vi "Gadgeton.vi"() -> ()   [LabVIEW 2019]
uses:
  <userlib>/_SmartBalloon/Balloon Generic/Aesthetics.ctl
  <userlib>/_SmartBalloon/API/Read Events.vi
  <userlib>/_SmartBalloon/Symbol Text Balloon/Symbol Text Balloon.lvclass
  C:/Program Files (x86)/National Instruments/LabVIEW 2019/user.lib/_SmartBalloon/Balloon Generic/Balloon.lvclass
  <vilib>/Utility/inputDevices.llb/closeKeyboard.vi
  <vilib>/Utility/inputDevices.llb/keyboardAcquire.vi
  <vilib>/Utility/inputDevices.llb/mouseAcquire.vi
  <vilib>/Utility/inputDevices.llb/closeMouse.vi
  <userlib>/_SmartBalloon/Balloon Generic/Balloon.lvclass
  <userlib>/_SmartBalloon/API/SmartBalloon Library.lvclass
panel:
  out "Grosss WPM":u64
  out "Present (s)":dbl
  out "Elapsed Time (s)":dbl
  in  "Time Target (s)":dbl=5.0
  out "Array":u64[](array[numeric])
  out "Waveform Chart - Dark":cluster{i16, dbl}(graph)
  in  "Stop Button":bool
  out "Mouse Button 1":bool
  out "Mouse Button 2":bool
  out "Horizontal Mouse Position":i32
  out "Vertical Mouse Position":i32
  out "Keys Pressed":T1(array[ring])
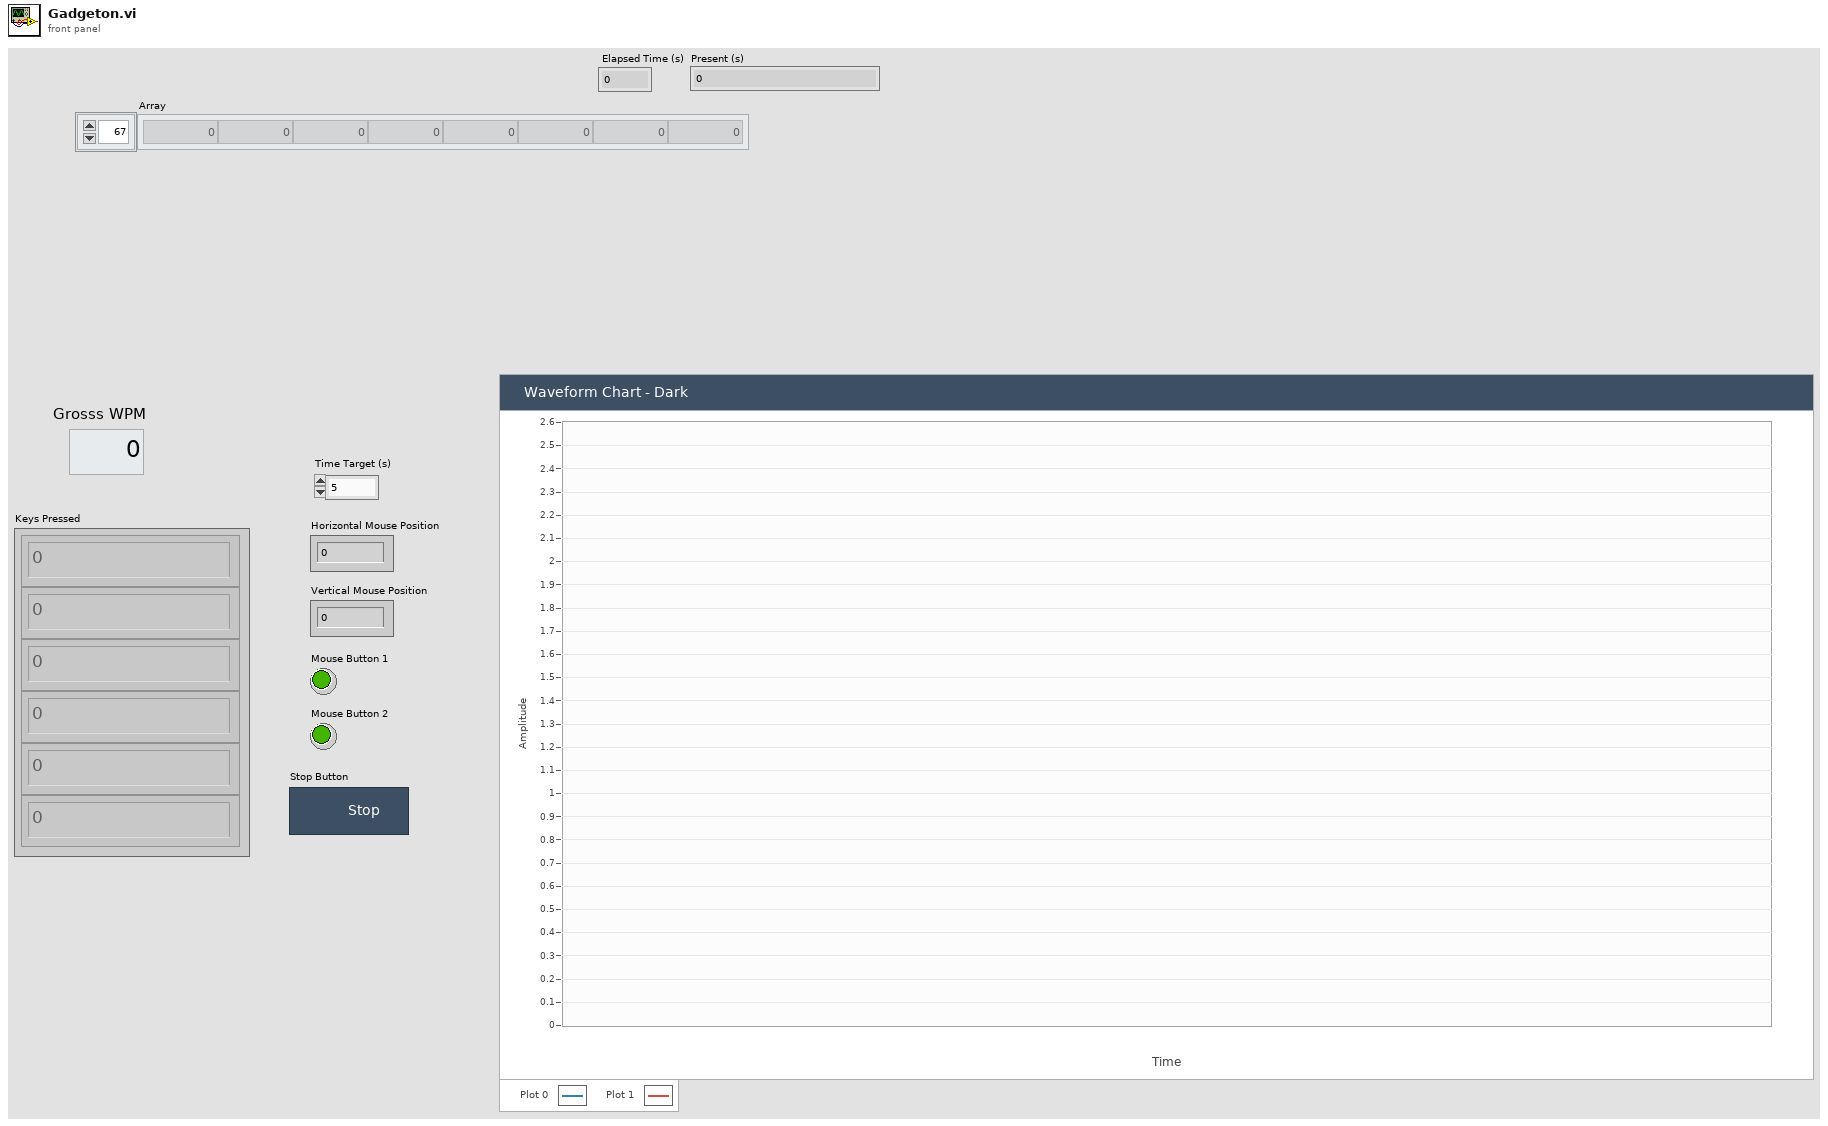
[diagram p1: front panel]
types:
  T1 = enum16{"0", "1", "2", "3", "4", "5", "6", "7", "8", "9", "A", "B", "C", "D", "E", "F", "G", "H", "I", "J", "K", "L", "M", "N", "O", "P", "Q", "R", "S", "T", "U", "V", "W", "X", "Y", "Z", "F1", "F2", "F3", "F4", "F5", "F6", "F7", "F8", "F9", "F10", "F11", "F12", "F13", "F14", "F15", "ADD", "BACK", "BACKSLASH", "CAPITAL", "COMMA", "DECIMAL", "DELETE", "DIVIDE", "DOWN", "END", "EQUALS", "ESCAPE", "GRAVE (`)", "HOME", "INSERT", "LBRACKET", "LCONTROL", "LEFT", "L ALT", "LSHIFT", "LWIN", "MINUS", "MULTIPLY", "NEXT", "NUMLOCK", "NUMPAD_0", "NUMPAD_1", "NUMPAD_2", "NUMPAD_3", "NUMPAD_4", "NUMPAD_5", "NUMPAD_6", "NUMPAD_7", "NUMPAD_8", "NUMPAD_9", "PAUSE", "PERIOD", "PRIOR (PG UP)", "RBRACKET", "RCONTROL", "RETURN", "RIGHT", "R ALT", "RSHIFT", "RWIN", "SCROLL", "SEMICOLON", "SLASH", "SPACE", "SUBTRACT", "TAB", "UP", "ENTER (num pad)", "' (quote)"}[]
  T2 = typedef "Balloon Engine.lvlib/Balloon.lvclass/Aesthetics.ctl" = cluster{"Colors":cluster{"Font Color":u32, "Panel Color":u32}, "Display Time (ms)":i32}
  T3 = cluster{"Horizontal":i32, "Vertical":i32, "Scrolling":i32}
  T4 = cluster{"button 1":bool, "button 2":bool, "button 3":bool, "button 4":bool}
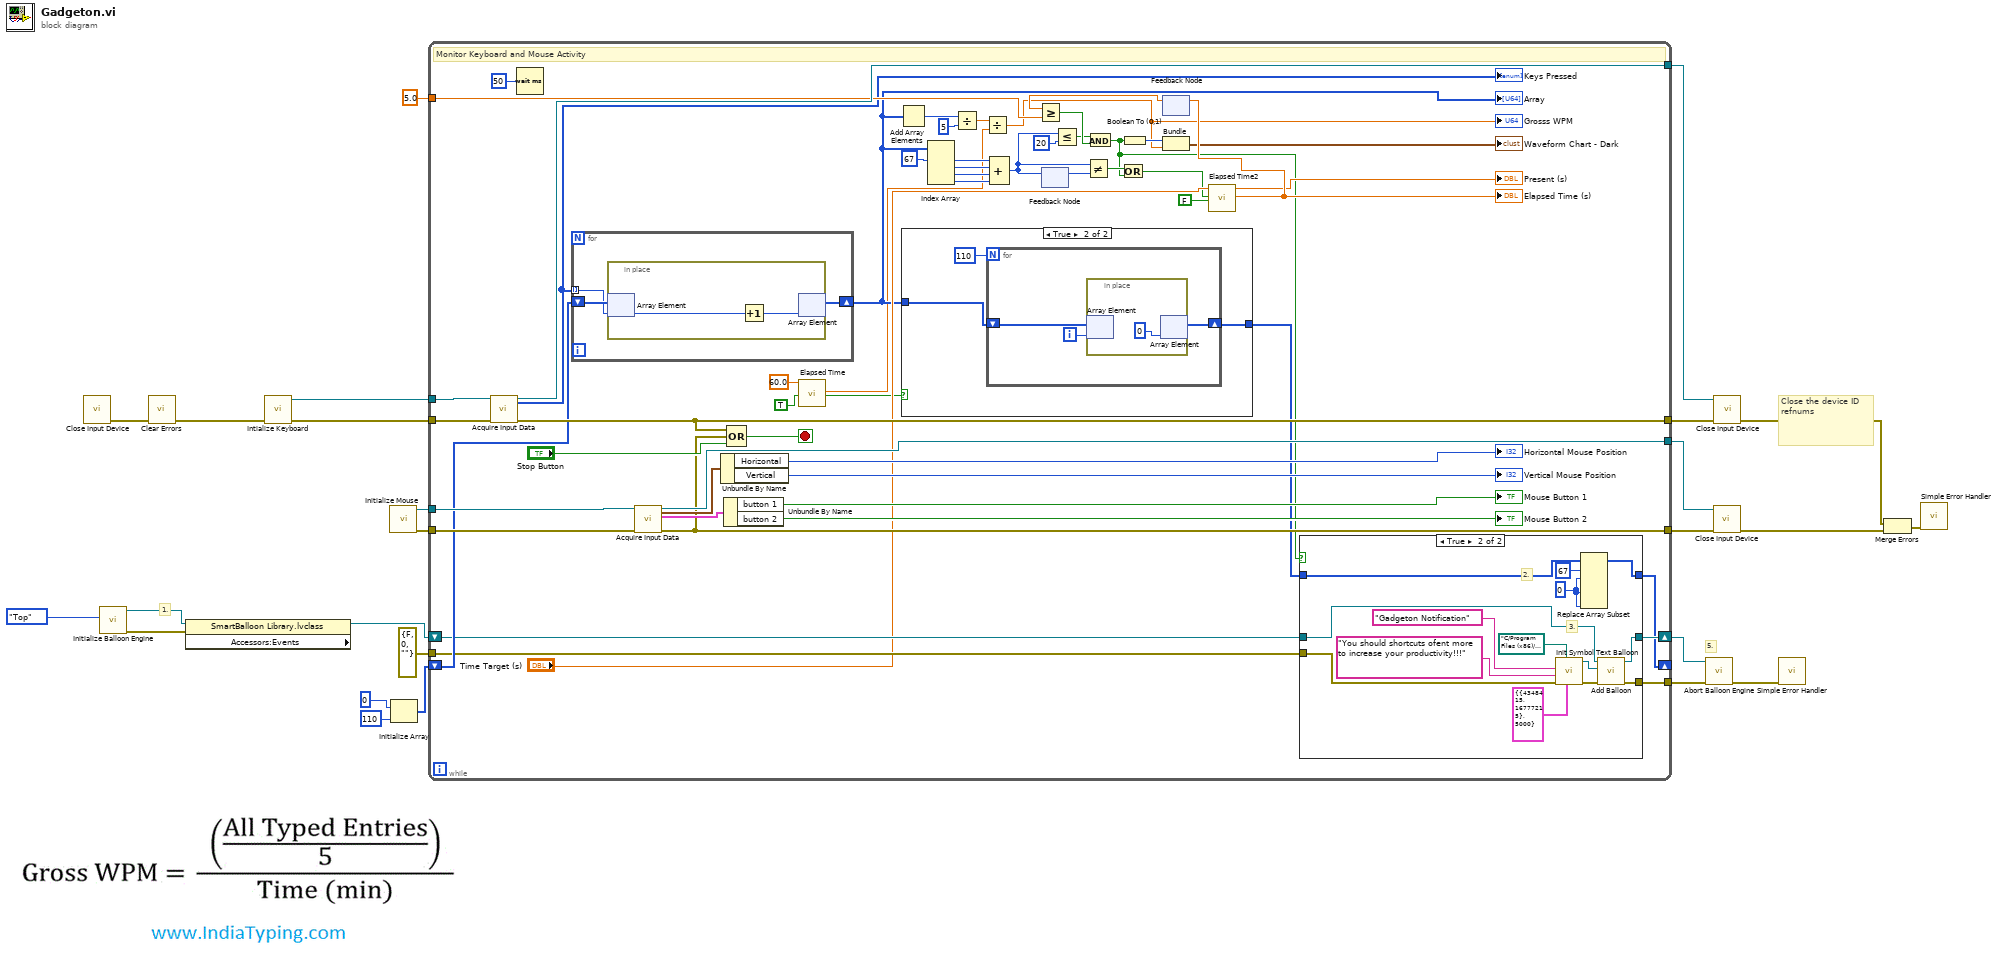
[diagram p0: block diagram]
diagram:
  # "5."
  # "1."
  # "Close the device ID refnums"
  n1 = call-poly <vilib>:"Close Input Device.vi"() -> ("error out"=w11:errorcluster)  [unwired: 2 in, 8 out]
  n2 = call <userlib>:"Initialize Balloon Engine.vi"("Balloon Direction"=enum16{"Top", "Bottom"}."Top" ("Balloon Position")) -> ("error out"=w9:errorcluster, "SmartBalloon Library.lvclass"=w8:refnum<class "SmartBalloon Library.lvclass">)  [unwired: 9 in]
  n3 = call <vilib>:"Clear Errors.vi"("error in (no error)"=w11) -> ("error out"=w10:errorcluster)  [unwired: 5 in, 1 out]
  n4 = property class="SmartBalloon Library.lvclass" props=["Accessors:Events"](reference=w8, error in=w9) -> (reference out=w6:refnum<class "SmartBalloon Library.lvclass">)  [unwired: 2 out]
  n5 = call <vilib>:"Intialize Keyboard.vi"("error in (no error)"=w10) -> ("error out"=w23:errorcluster, "device ID"=w25:refnum<k1>)  [unwired: 9 out]
  n6 = call <vilib>:"Initialize Mouse.vi"() -> ("error out"=w22:errorcluster, "device ID"=w24:refnum<k1>)  [unwired: 1 in, 9 out]
  n7 = Initialize Array(u64 0, 110 ("dimension size")) -> (w12:u64[])
  n8 = while {
    tunnel: [w65] -> w17
    tunnel: [w74] -> w18
    tunnel: [w64] -> w19
    tunnel: w22 -> [w78]
    tunnel: w23 -> [w79]
    tunnel: w24 -> [w80]
    tunnel: [w75] -> w20
    tunnel: w25 -> [w73]
    shift-right: [w40] -> _
    shift-left: w12 -> [w63]
    shift-right: [w53] -> w4
    shift-left: w6 -> [w54]
    tunnel: errorcluster {"status"=FALSE, "code"=0, "source"=""} ("error out") -> [w52]
    tunnel: [w51] -> w3
    tunnel: 5.0 ("y") -> [w50]
    stop <- w66 stop-if-true
    # "Monitor Keyboard and Mouse Activity"
    n9 = call-poly <vilib>:"Acquire Input Data.vi"("device ID"=w73, "error in (no error)"=w79) -> ("device ID"=w75:refnum<k1>, "keys pressed"=w38:T1, "error out"=w64:errorcluster)  [unwired: 15 out]
    "Keys Pressed" <- w38
    n10 = Wait (ms)(milliseconds to wait=u32 50) -> ()  [unwired: 1 out]
    n11 = for {
      tunnel: w38 -> [w107] mode=indexing
      shift-right: [w106] -> w34
      shift-left: w63 -> [w108]
      n12 = in-place {
        n13 = in-place-array #1(w108, w107) -> (w110:u64)
        n14 = Increment(x=w110) -> (x+1=w109:u64)
        n15 = in-place-array #1(w109) -> (w106:u64[])  [unwired: 1 out]
      }
    }
    "Array" <- w34
    n16 = call-poly <vilib>:"Acquire Input Data.vi"("device ID"=w80, "error in (no error)"=w78) -> ("device ID"=w74:refnum<k1>, "axis info"=w70:T3, "button info"=w77:T4, "error out"=w65:errorcluster)  [unwired: 1 in, 13 out]
    n17 = Unbundle By Name(w70) -> ("Horizontal"=→"Horizontal Mouse Position":i32, "Vertical"=→"Vertical Mouse Position":i32)
    n18 = Unbundle By Name(w77) -> ("button 1"=→"Mouse Button 1":bool, "button 2"=→"Mouse Button 2":bool)
    n19 = Compound Arithmetic op=OR(w64, w65, "Stop Button") -> (w66:bool)
    n20 = call "Elapsed Time"("Time Target (s)"=60.0, "Auto Reset"=TRUE) -> ("Elapsed Time (s)"=w30:dbl, "Time has Elapsed"=w36:bool)  [unwired: 10 in, 6 out]
    n21 = Add Array Elements(numeric array=w34) -> (sum=w32:u64)
    n22 = case shown="True" w36 {
      tunnel: w34 -> [w81 w82]
      tunnel: [w81 w84] -> w35
      frame False {
      }
      frame True {
        n23 = for {
          N: 110 -> [_]
          shift-right: [w85] -> w84
          shift-left: w82 -> [w87]
          i -> [w86]
          n24 = in-place {
            n25 = in-place-array #2(w87, w86) -> ()  [unwired: 1 out]
            n26 = in-place-array #2(u64 0 ("element")) -> (w85:u64[])  [unwired: 1 out]
          }
        }
      }
    }
    n27 = Index Array(array=w34, index #1=67 ("index")) -> (element #1=w61:u64, element #2=w60:u64, element #3=w59:u64, element #4=w58:u64)  [unwired: 3 in]
    n28 = Divide(x=w32, y=u64 5) -> (x/y=w33:dbl)
    n29 = Divide(x=w33, y=w30) -> (x/y=w27:dbl)
    "Grosss WPM" <- w27
    n30 = Compound Arithmetic op=ADD(w61, w60, w59, w58) -> (w47:u64)
    n31 = feedback-in #3(w47) -> ()
    n32 = feedback #3() -> (w46:u64)  [unwired: 1 in]
    n33 = Less Or Equal?(x=w47, y=u64 20) -> (x <= y?=w55:bool)
    n34 = Not Equal?(x=w47, y=w46) -> (x != y?=w45:bool)
    n35 = feedback #4() -> (w42:dbl)  [unwired: 1 in]
    n36 = Greater Or Equal?(x=w42, y=w50) -> (x >= y?=w57:bool)
    n37 = And(x=w55, y=w57) -> (x .and. y?=w39:bool)
    n38 = Or(x=w45, y=w39) -> (x .or. y?=w44:bool)
    n39 = Boolean To (0,1)(Boolean=w39) -> (0, 1=w28:i16)
    n40 = Bundle(w28, w27) -> (→"Waveform Chart - Dark":cluster{i16, dbl})  [unwired: 1 in]
    n41 = call "Elapsed Time2"("Time Target (s)"="Time Target (s)", "Reset"=w44, "Auto Reset"=FALSE) -> ("Present (s)"=→"Present (s)":dbl, "Elapsed Time (s)"=w43:dbl)  [unwired: 9 in, 6 out]
    "Elapsed Time (s)" <- w43
    n42 = feedback-in #4(w43) -> ()
    n43 = case shown="True" w39 {
      tunnel: w54 -> [w91 w105]
      tunnel: [w91 w104] -> w53
      tunnel: w52 -> [w90 w103]
      tunnel: [w90 w102] -> w51
      tunnel: [w89 w93] -> w40
      tunnel: w35 -> [w89 w92]
      frame False {
      }
      frame True {
        w94 = u64 0 ("new element/subarray")
        # "3."
        # "2."
        n44 = call <userlib>:"Init Symbol Text Balloon.vi"("Aesthetics"=T2 {"Colors"={"Font Color"=4348415, "Panel Color"=16777215}, "Display Time (ms)"=5000} ("Balloon Settings"), "Symbol File Name"=path "C:/Program Files (x86)/National Instruments/LabVIEW 2019/examples/SmartBalloon/Icons/info.png", "error in (no error)"=w103, "Body"="You should shortcuts ofent more to increase your productivity!!!", "Title"="Gadgeton Notification") -> ("error out"=w97:errorcluster, "Symbol Text Balloon out"=w96:refnum<class "Symbol Text Balloon.lvclass">)  [unwired: 5 in]
        n45 = Replace Array Subset(array=w92, new element #1=w94, index #1=67 ("index"), new element #2=w94, new element #3=w94) -> (w93:u64[])  [unwired: 2 in]
        n46 = call <userlib>:"Add Balloon.vi"("error in (no error)"=w97, "Next Balloon"=w96, "SmartBalloon Engine Reference"=w105) -> ("error out"=w102:errorcluster, "SmartBalloon Engine Reference out"=w104:refnum<class "SmartBalloon Library.lvclass">)  [unwired: 7 in]
      }
    }
  }
  n47 = call <userlib>:"Abort Balloon Engine.vi"("error in (no error)"=w3, "SmartBalloon Engine Reference"=w4) -> ("error out"=w1:errorcluster)  [unwired: 9 in]
  n48 = call-poly <vilib>:"Close Input Device.vi"("error in (no error)"=w17, "device ID"=w18) -> ("error out"=w16:errorcluster)  [unwired: 8 out]
  n49 = call-poly <vilib>:"Close Input Device.vi"("error in (no error)"=w19, "device ID"=w20) -> ("error out"=w15:errorcluster)  [unwired: 8 out]
  n50 = call <vilib>:"Simple Error Handler.vi"("error in (no error)"=w1) -> ()  [unwired: 4 in, 5 out]
  n51 = Merge Errors(w15, w16) -> (w21:errorcluster)
  n52 = call <vilib>:"Simple Error Handler.vi"("error in (no error)"=w21) -> ()  [unwired: 4 in, 5 out]
